vi "Global PhaseStandalone.vi"() -> ()   [LabVIEW 2011]
panel:
  out "Beadlist done!":bool
  out "Stop all":bool
  out "Tuned Phase tracker":bool
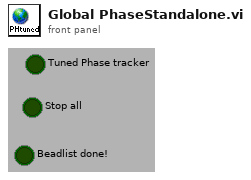
[diagram p1: front panel]
diagram:
